vi "Get Data.vi"(8 "error in":errorcluster, 11 "PAS UI In":refnum<class "PAS UI.lvclass">) -> (0 "error out":errorcluster, 1 "Stop?":bool, 2 "Data":refnum<class "Data.lvclass">, 3 "PAS UI Out":refnum<class "PAS UI.lvclass">)   [LabVIEW 2012, in "PAS UI.lvclass"]
uses:
  Generic UI/PAS UI.lvclass
  Reusable/GUI/GUI.lvclass
  Reusable/Data/Data.lvclass
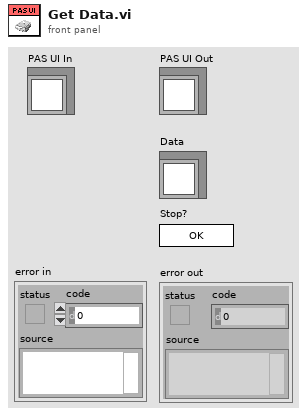
[diagram p1: front panel]
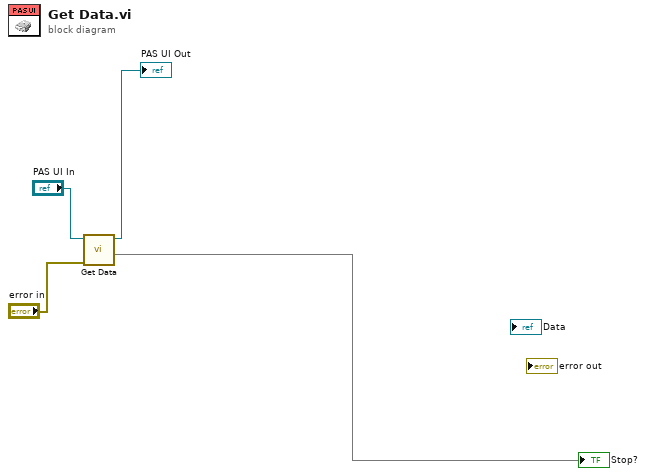
[diagram p0: block diagram]
diagram:
  n1 = call-parent "Get Data.vi"("error in"="error in", "GUI in"="PAS UI In") -> (1:→"Stop?", "GUI out"=→"PAS UI Out":refnum<class "PAS UI.lvclass">)  [unwired: 6 in, 2 out]
